vi "FABR-Process Frame.vi"(0 "Runtime in":T3, 5 "Tickets in":T1[](array[typedef]), 7 "SCL in":T2[](array[typedef]), 9 "AI Waveforms":dbl[](array[numeric]), 11 "error in (no error)":errorcluster, 12 "Reject":dbl, 13 "override":bool) -> (2 "reject fraction":dbl, 3 "Raw":dbl[](array[numeric]), 4 "Runtime out":T3, 6 "Tickets out":T1[](array[typedef]), 8 "SCL out":T2[](array[typedef]), 10 "update":T2[](array[typedef]), 15 "error out":errorcluster)   [LabVIEW 2020]
uses:
  Typedefs/FABR-Stimulus Condition.ctl
  Typedefs/FABR-Runtime Data.ctl
  Typedefs/FABR-Stimulus Ticket.ctl
  <vilib>/Analysis/baseanly.llb/Mean.vi
  <vilib>/Analysis/baseanly.llb/Mean (DBL).vi
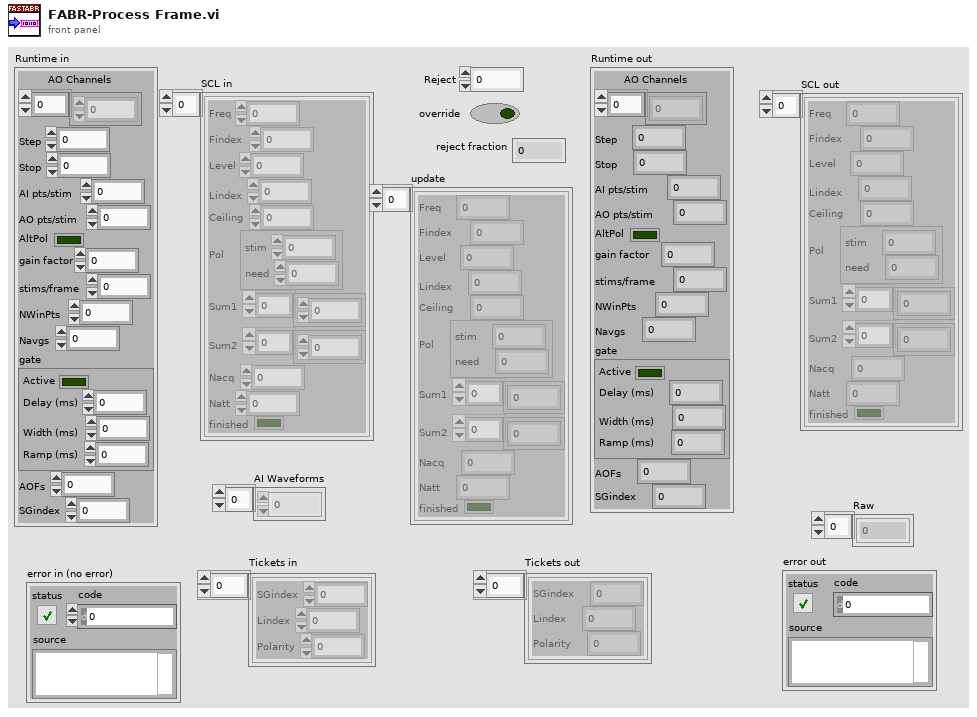
[diagram p1: front panel]
types:
  T1 = typedef "FABR-Stimulus Ticket.ctl" = cluster{"SGindex":i32, "Lindex":i32, "Polarity":i32}
  T2 = typedef "FABR-Stimulus Condition.ctl" = cluster{"Freq":dbl, "Findex":i32, "Level":dbl, "Lindex":i32, "Ceiling":dbl, "Pol":cluster{"stim":i32, "need":i32}, "Sum1":dbl[], "Sum2":dbl[], "Nacq":i32, "Natt":i32, "finished":bool}
  T3 = typedef "FABR-Runtime Data.ctl" = cluster{"AO Channels":i32[], "Step":dbl, "Stop":i32, "AI pts/stim":i32, "AO pts/stim":i32, "AltPol":bool, "gain factor":dbl, "stims/frame":i32, "NWinPts":i32, "Navgs":i32, "gate":cluster{"Active":bool, "Delay (ms)":dbl, "Width (ms)":dbl, "Ramp (ms)":dbl}, "AOFs":dbl, "SGindex":i32}
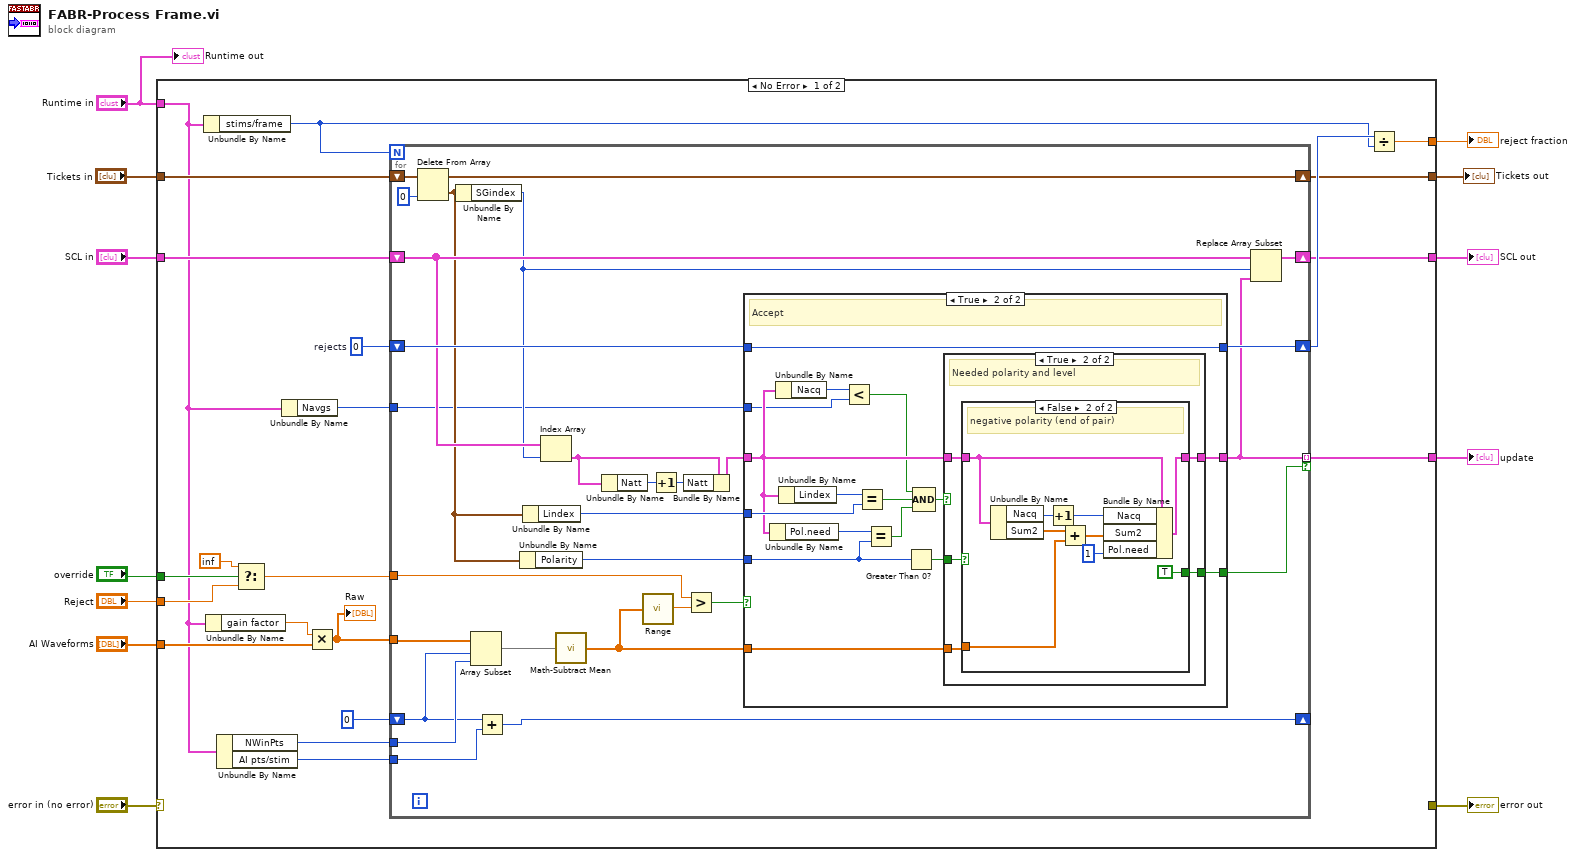
[diagram p0: block diagram]
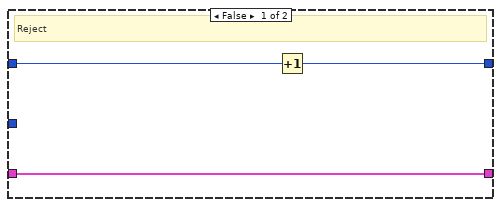
[diagram p2: hidden frame]
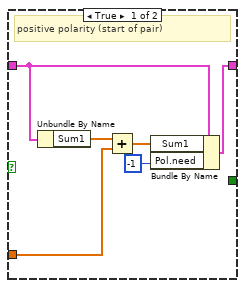
[diagram p4: hidden frame]
diagram:
  n1 = case shown="No Error" "error in (no error)" {
    selector: "error in (no error)" -> [_ w103]
    tunnel: "Runtime in" -> [w14 _]
    tunnel: "AI Waveforms" -> [w33 _]
    tunnel: "override" -> [w27 _]
    tunnel: "Reject" -> [w26 _]
    tunnel: "SCL in" -> [w16 _]
    tunnel: [w20 _] -> w7
    tunnel: [w19 _] -> w6
    tunnel: [w18 _] -> w5
    tunnel: [_ w103] -> w4
    tunnel: "Tickets in" -> [w17 w102]
    tunnel: [w15 w102] -> w1
    frame No Error {
      w23 = 0  # rejects
      n2 = Unbundle By Name(w14) -> ("stims/frame"=w21:i32)
      n3 = Unbundle By Name(w14) -> ("gain factor"=w32:dbl)
      n4 = Unbundle By Name(w14) -> ("NWinPts"=w29:i32, "AI pts/stim"=w28:i32)
      n5 = Select(t=inf, s=w27, f=w26) -> (s? t:f=w24:dbl)
      n6 = Unbundle By Name(w14) -> ("Navgs"=w13:i32)
      n7 = Multiply(x=w32, y=w33) -> (x*y=w31:dbl[])
      "Raw" <- w31
      n8 = for {
        N: w21 -> [_]
        tunnel: w31 -> [w61]
        shift-right: [w57] -> _
        shift-left: 0 -> [w59]
        tunnel: w29 -> [w60]
        tunnel: w28 -> [w58]
        tunnel: w24 -> [w54]
        shift-right: [w51] -> w22
        shift-left: w23 -> [w50]
        shift-right: [w44] -> w18
        shift-left: w16 -> [w45]
        tunnel: [w43] -> w19 mode=indexing if=w42
        shift-right: [w40] -> w15
        shift-left: w17 -> [w41]
        tunnel: w13 -> [w35]
        n9 = Delete From Array(array=w41, index=0) -> (deleted portion=w37:T1, array with subset deleted=w40:T1[])  [unwired: 1 in]
        n10 = Unbundle By Name(w37) -> ("SGindex"=w39:i32)
        n11 = Array Subset(array=w61, index=w59, length=w60) -> (w56:dbl[])
        n12 = Add(x=w59, y=w58) -> (x+y=w57:i32)
        n13 = Unbundle By Name(w37) -> ("Polarity"=w36:i32)
        n14 = Unbundle By Name(w37) -> ("Lindex"=w38:i32)
        n15 = Index Array(array=w45, index=w39) -> (element=w47:T2)
        n16 = call "Math-Subtract Mean.vi"("Y"=w56) -> ("Y - mean(Y)"=w52:dbl[])  [unwired: 4 in]
        n17 = Unbundle By Name(w47) -> ("Natt"=w49:i32)
        n18 = call "Range.vi"("Array"=w52) -> ("Range"=w55:dbl)
        n19 = Increment(x=w49) -> (x+1=w48:i32)
        n20 = Bundle By Name(cluster=w47, "Natt"=w48) -> (w46:T2)
        n21 = Greater?(x=w54, y=w55) -> (0:w53:bool)
        n22 = case shown="True" w53 {
          tunnel: w52 -> [_ w78]
          tunnel: [w63 w80] -> w51
          tunnel: w50 -> [w64 w80]
          tunnel: w46 -> [w62 w67]
          tunnel: [w62 w77] -> w43
          tunnel: [_ w76] -> w42
          tunnel: w36 -> [_ w74]
          tunnel: w38 -> [_ w73]
          tunnel: w35 -> [_ w66]
          frame False {
            # "Reject"
            n23 = Increment(x=w64) -> (x+1=w63:i32)
          }
          frame True {
            # "Accept"
            n24 = Unbundle By Name(w67) -> ("Pol.need"=w75:i32)
            n25 = Unbundle By Name(w67) -> ("Nacq"=w68:i32)
            n26 = Unbundle By Name(w67) -> ("Lindex"=w72:i32)
            n27 = Less?(x=w68, y=w66) -> (x < y?=w65:bool)
            n28 = Equal?(x=w72, y=w73) -> (x = y?=w70:bool)
            n29 = Equal?(x=w75, y=w74) -> (x = y?=w71:bool)
            n30 = Greater Than 0?(x=w74) -> (x > 0?=w79:bool)
            n31 = Compound Arithmetic op=AND(w65, w70, w71) -> (w69:bool)
            n32 = case shown="True" w69 {
              tunnel: w79 -> [_ w86]
              tunnel: w78 -> [_ w85]
              tunnel: w67 -> [w81 w84]
              tunnel: [w81 w83] -> w77
              tunnel: [_ w82] -> w76
              frame False {
                # "Wrong polarity or level"
              }
              frame True {
                # "Needed polarity and level"
                n33 = case shown="False" w86 {
                  tunnel: w84 -> [w89 w99]
                  tunnel: w85 -> [w91 w100]
                  tunnel: [w88 w95] -> w83
                  tunnel: [_ TRUE] -> w82
                  frame True {
                    # "positive polarity (start of pair)"
                    n34 = Unbundle By Name(w89) -> ("Sum1"=w92:dbl[])
                    n35 = Add(x=w92, y=w91) -> (x+y=w90:dbl[])
                    n36 = Bundle By Name(cluster=w89, "Sum1"=w90, "Pol.need"=-1 ("awaiting")) -> (w88:T2)
                  }
                  frame False {
                    # "negative polarity (end of pair)"
                    n37 = Unbundle By Name(w99) -> ("Nacq"=w97:i32, "Sum2"=w101:dbl[])
                    n38 = Increment(x=w97) -> (x+1=w96:i32)
                    n39 = Add(x=w101, y=w100) -> (x+y=w98:dbl[])
                    n40 = Bundle By Name(cluster=w99, "Nacq"=w96, "Sum2"=w98, "Pol.need"=1 ("awaiting")) -> (w95:T2)
                  }
                }
              }
            }
          }
        }
        n41 = Replace Array Subset(array=w45, new element=w43, index=w39) -> (w44:T2[])
      }
      n42 = Divide(x=w22, y=w21) -> (x/y=w20:dbl)
    }
    frame Error {
    }
  }
  "error out" <- w4
  "SCL out" <- w5
  "update" <- w6
  "reject fraction" <- w7
  "Tickets out" <- w1
  "Runtime out" <- "Runtime in"
